vi "Send Items To Target.vi"(8 "error in (no error)":errorcluster, 9 "TransferOptions":refnum<class "FileTransferOptions.lvclass">, 10 "FileTransfer":refnum<class "FileTransfer.lvclass">, 11 "Session in":refnum<class "Session.lvclass">) -> (0 "error out":errorcluster, 2 "Transfer Status":T3, 3 "Session out":refnum<class "Session.lvclass">)   [LabVIEW 2015, in "WinSCP.lvlib" / "Session.lvclass"]
uses:
  Session.lvclass
  FileTransfer/FileTransfer.lvclass
  FileTransferOptions/FileTransferOptions.lvclass
  FileTransfer/FileAndDestination.ctl
  FileTransfer/TransferExceptionDescription.ctl
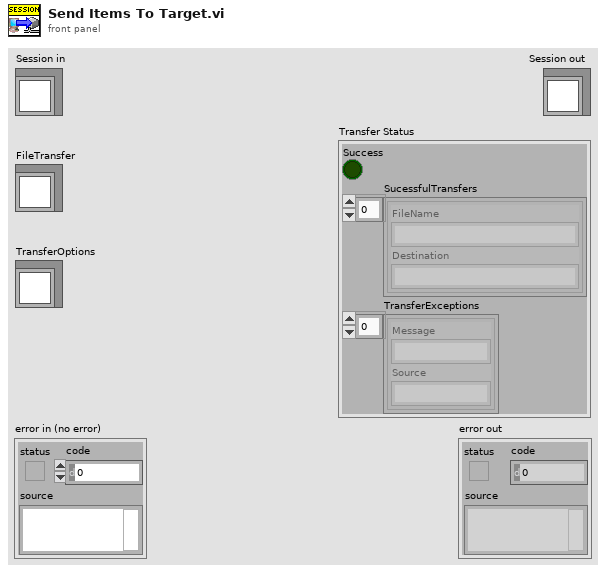
[diagram p1: front panel]
types:
  T1 = typedef "WinSCP.lvlib/FileTransfer.lvclass/FileAndDestination.ctl" = cluster{"FileName":string, "Destination":string}
  T2 = typedef "WinSCP.lvlib/FileTransfer.lvclass/TransferExceptionDescription.ctl" = cluster{"Message":string, "Source":string}
  T3 = cluster{"Success":bool, "SucessfulTransfers":T1[], "TransferExceptions":T2[]}
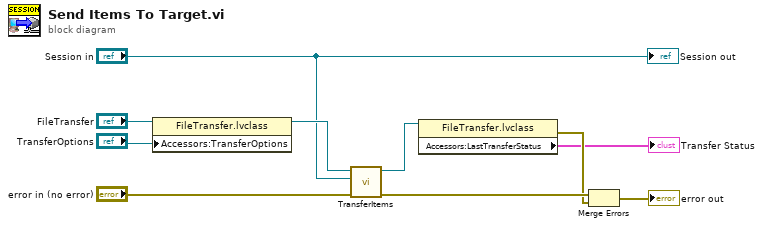
[diagram p0: block diagram]
diagram:
  n1 = property class="FileTransfer.lvclass"(reference="FileTransfer", "Accessors:TransferOptions"="TransferOptions") -> (reference out=w8:refnum<class "FileTransfer.lvclass">)  [unwired: 1 in, 1 out]
  n2 = call-dynamic "TransferItems.vi"("error in (no error)"="error in (no error)", "Session"="Session in", "FileTransfer in"=w8) -> ("error out"=w10:errorcluster, "FileTransfer out"=w9:refnum<class "FileTransfer.lvclass">)  [unwired: 7 in]
  n3 = property class="FileTransfer.lvclass"(reference=w9) -> (error out=w7:errorcluster, "Accessors:LastTransferStatus"=→"Transfer Status":T3)  [unwired: 1 in, 1 out]
  n4 = Merge Errors(w10, w7) -> (→"error out":errorcluster)
  "Session out" <- "Session in"
